vi "Listen for Network Broadcasts.vi"(6 "Local IP Address":string, 7 "Max Rx Byte Size":i32, 8 "error in (no error)":errorcluster, 9 "Port":u16, 10 "Multicast Address":string, 11 "Module ID":i32=-1) -> (0 "error out":errorcluster)   [LabVIEW 2014, in "GenNet-Client.lvlib"]
doc: "Opens a port to listen for broadcasts sent by other modules via UDP\n_____\nCreated using Delacor QMH Event Scripter 4.2.1.88."
uses:
  GenNet-Client.lvlib
  Listen for Network Broadcasts Argument--cluster.ctl
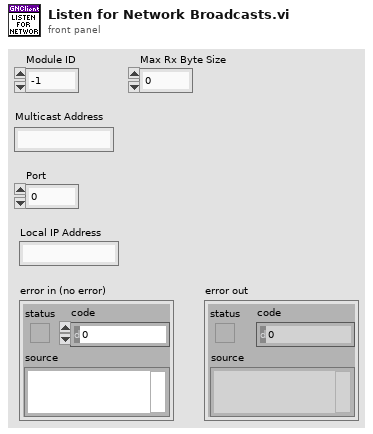
[diagram p1: front panel]
types:
  T1 = typedef "GenNet-Client.lvlib/Listen for Network Broadcasts Argument--cluster.ctl" = cluster{"Module ID":i32, "Multicast Address":string, "Port":u16, "Local IP Address":string, "Max Rx Byte Size":i32}
  T2 = typedef "GenNet-Client.lvlib/Request Events--cluster.ctl" = cluster{"Stop Module":refnum<user-event>, "Show Panel":refnum<user-event>, "Hide Panel":refnum<user-event>, "Show Diagram":refnum<user-event>, "Get Module Execution Status":refnum<user-event>, "Send via Network":refnum<user-event>, "Connect":refnum<user-event>, "Listen for Network Broadcasts":refnum<user-event>}
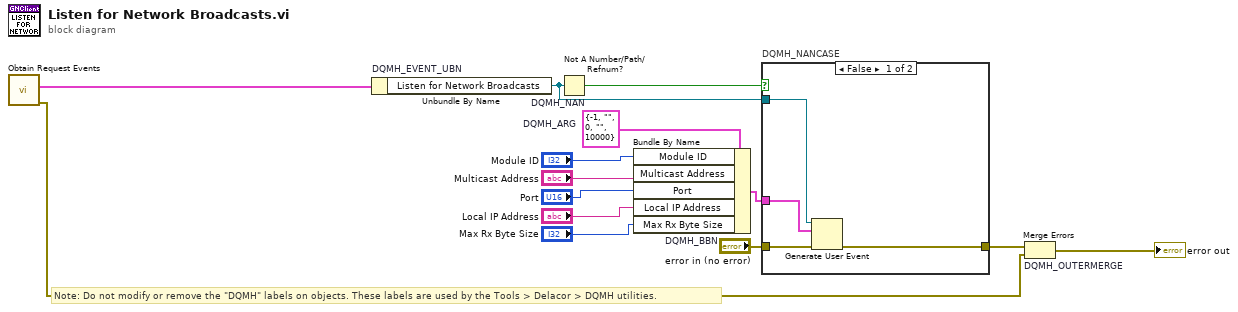
[diagram p0: block diagram]
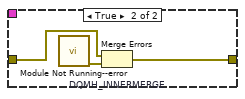
[diagram p2: hidden frame]
diagram:
  w8 = T1 {"Module ID"=-1, "Multicast Address"="", "Port"=0, "Local IP Address"="", "Max Rx Byte Size"=10000}  # DQMH_ARG
  # "Note: Do not modify or remove the \"DQMH\" labels on objects. These labels are used by the Tools > Delacor > DQMH utilities."
  n1 = call "Obtain Request Events.vi"() -> ("error out"=w4:errorcluster, "GenNet-Client Request Events"=w3:T2)  [unwired: 10 in]
  n2 = Unbundle By Name "DQMH_EVENT_UBN"(w3) -> ("Listen for Network Broadcasts"=w10:refnum<user-event>)
  n3 = Not A Number/Path/Refnum? "DQMH_NAN"(number/path/refnum=w10) -> (NaN/Path/Refnum?=w11:bool)
  n4 = Bundle By Name "DQMH_BBN"(cluster=w8, "Module ID"="Module ID", "Multicast Address"="Multicast Address", "Port"="Port", "Local IP Address"="Local IP Address", "Max Rx Byte Size"="Max Rx Byte Size") -> (w12:T1)
  n5 = case "DQMH_NANCASE" shown="False" w11 {
    tunnel: "error in (no error)" -> [w18 w21]
    tunnel: [w17 w20] -> w9
    tunnel: w10 -> [w16 _]
    tunnel: w12 -> [w15 _]
    frame False {
      n6 = Generate User Event(user event=w16, event data cluster=w15, error in=w18) -> (error out=w17:errorcluster)  [unwired: 1 in, 1 out]
    }
    frame True {
      n7 = call "Module Not Running--error.vi"() -> ("error out"=w19:errorcluster)  [unwired: 11 in]
      n8 = Merge Errors "DQMH_INNERMERGE"(w21, w19) -> (w20:errorcluster)
    }
  }
  n9 = Merge Errors "DQMH_OUTERMERGE"(w9, w4) -> (→"error out":errorcluster)
